vi "WriteIOSafeCondition gas.vi"(1 "error in":errorcluster) -> (0 "error out":errorcluster)   [LabVIEW 2011]
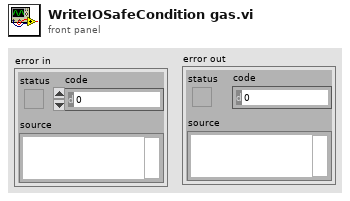
[diagram p1: front panel]
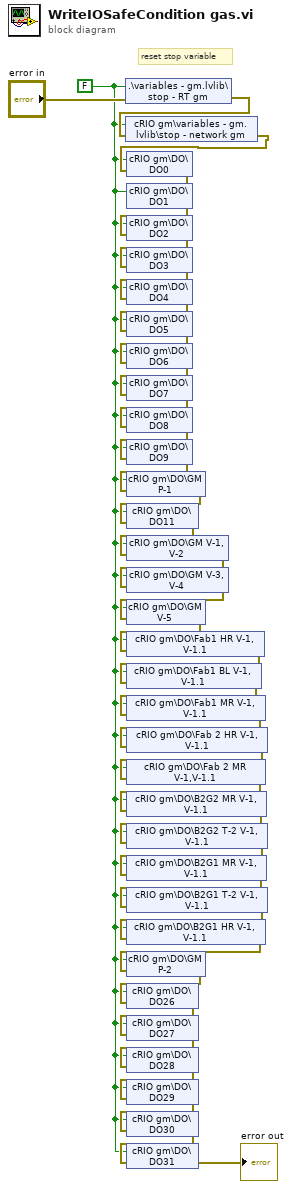
[diagram p0: block diagram]
diagram:
  w1 = FALSE ("B2G1 P-4")
  # "reset stop variable"
  n1 = shared-variable ".\\variables - gm.lvlib\\stop - RT gm"(w1, error in="error in") -> (error out=w35:errorcluster)
  n2 = shared-variable "cRIO gm\\variables - gm.lvlib\\stop - network gm"(w1, error in=w35) -> (error out=w34:errorcluster)
  n3 = shared-variable "cRIO gm\\DO\\DO0"(w1, error in=w34) -> (error out=w33:errorcluster)
  n4 = shared-variable "cRIO gm\\DO\\DO1"(w1, error in=w33) -> (error out=w2:errorcluster)
  n5 = shared-variable "cRIO gm\\DO\\DO2"(w1, error in=w2) -> (error out=w3:errorcluster)
  n6 = shared-variable "cRIO gm\\DO\\DO3"(w1, error in=w3) -> (error out=w4:errorcluster)
  n7 = shared-variable "cRIO gm\\DO\\DO4"(w1, error in=w4) -> (error out=w5:errorcluster)
  n8 = shared-variable "cRIO gm\\DO\\DO5"(w1, error in=w5) -> (error out=w6:errorcluster)
  n9 = shared-variable "cRIO gm\\DO\\DO6"(w1, error in=w6) -> (error out=w7:errorcluster)
  n10 = shared-variable "cRIO gm\\DO\\DO7"(w1, error in=w7) -> (error out=w8:errorcluster)
  n11 = shared-variable "cRIO gm\\DO\\DO8"(w1, error in=w8) -> (error out=w9:errorcluster)
  n12 = shared-variable "cRIO gm\\DO\\DO9"(w1, error in=w9) -> (error out=w10:errorcluster)
  n13 = shared-variable "cRIO gm\\DO\\GM P-1"(w1, error in=w10) -> (error out=w11:errorcluster)
  n14 = shared-variable "cRIO gm\\DO\\DO11"(w1, error in=w11) -> (error out=w12:errorcluster)
  n15 = shared-variable "cRIO gm\\DO\\GM V-1, V-2"(w1, error in=w12) -> (error out=w13:errorcluster)
  n16 = shared-variable "cRIO gm\\DO\\GM V-3, V-4"(w1, error in=w13) -> (error out=w14:errorcluster)
  n17 = shared-variable "cRIO gm\\DO\\GM V-5"(w1, error in=w14) -> (error out=w15:errorcluster)
  n18 = shared-variable "cRIO gm\\DO\\Fab1 HR V-1, V-1.1"(w1, error in=w15) -> (error out=w16:errorcluster)
  n19 = shared-variable "cRIO gm\\DO\\Fab1 BL V-1, V-1.1"(w1, error in=w16) -> (error out=w17:errorcluster)
  n20 = shared-variable "cRIO gm\\DO\\Fab1 MR V-1, V-1.1"(w1, error in=w17) -> (error out=w18:errorcluster)
  n21 = shared-variable "cRIO gm\\DO\\Fab 2 HR V-1, V-1.1"(w1, error in=w18) -> (error out=w19:errorcluster)
  n22 = shared-variable "cRIO gm\\DO\\Fab 2 MR V-1,V-1.1"(w1, error in=w19) -> (error out=w20:errorcluster)
  n23 = shared-variable "cRIO gm\\DO\\B2G2 MR V-1, V-1.1"(w1, error in=w20) -> (error out=w21:errorcluster)
  n24 = shared-variable "cRIO gm\\DO\\B2G2 T-2 V-1, V-1.1"(w1, error in=w21) -> (error out=w22:errorcluster)
  n25 = shared-variable "cRIO gm\\DO\\B2G1 MR V-1, V-1.1"(w1, error in=w22) -> (error out=w23:errorcluster)
  n26 = shared-variable "cRIO gm\\DO\\B2G1 T-2 V-1, V-1.1"(w1, error in=w23) -> (error out=w24:errorcluster)
  n27 = shared-variable "cRIO gm\\DO\\B2G1 HR V-1, V-1.1"(w1, error in=w24) -> (error out=w25:errorcluster)
  n28 = shared-variable "cRIO gm\\DO\\GM P-2"(w1, error in=w25) -> (error out=w26:errorcluster)
  n29 = shared-variable "cRIO gm\\DO\\DO26"(w1, error in=w26) -> (error out=w27:errorcluster)
  n30 = shared-variable "cRIO gm\\DO\\DO27"(w1, error in=w27) -> (error out=w28:errorcluster)
  n31 = shared-variable "cRIO gm\\DO\\DO28"(w1, error in=w28) -> (error out=w29:errorcluster)
  n32 = shared-variable "cRIO gm\\DO\\DO29"(w1, error in=w29) -> (error out=w30:errorcluster)
  n33 = shared-variable "cRIO gm\\DO\\DO30"(w1, error in=w30) -> (error out=w31:errorcluster)
  n34 = shared-variable "cRIO gm\\DO\\DO31"(w1, error in=w31) -> (error out=→"error out":errorcluster)
